vi "publish -- write -- num.vi"(8 "request event":refnum<user-event>, 9 "response in":refnum<user-event>, 11 "Numeric":dbl format="%#_13g") -> (1 "response out":refnum<user-event>)   [LabVIEW 2018]
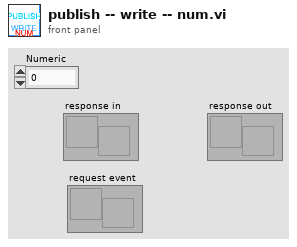
[diagram p1: front panel]
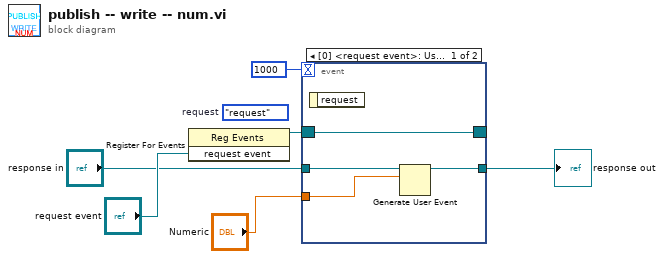
[diagram p0: block diagram]
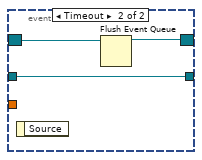
[diagram p2: hidden frame]
diagram:
  (unwired) enum16{"request"}."request"  # request
  n1 = register-events("request event") -> (reference out=w6:refnum<event-registration>)  [unwired: 2 in, 1 out]
  n2 = event shown="[0] <request event>: User Event" {
    selector: w6 -> [w10 w13]
    dyn-events: [w10 w12] -> _
    timeout: 1000 -> [_ _]
    tunnel: "response in" -> [w9 w11]
    tunnel: "Numeric" -> [w8 _]
    tunnel: [w7 w11] -> w1
    event User Event {
      n3 = event-data() -> ()  [unwired: 1 in, 1 out]
      n4 = Generate User Event(user event=w9, event data cluster=w8) -> (user event out=w7:refnum<user-event>)  [unwired: 2 in, 1 out]
    }
    event Timeout {
      n5 = event-data() -> ()  [unwired: 1 in, 1 out]
      n6 = Flush Event Queue(0:w13) -> (8:w12:refnum<event-registration>)  [unwired: 5 in, 2 out]
    }
  }
  "response out" <- w1
